vi "about status.vi"(8 "error in (no error)":errorcluster, 11 "Connection Refnum":T1) -> (0 "error out":errorcluster, 3 "Keys":T2)   [LabVIEW 2011]
uses:
  ITK EXT/utils/keyedarr.llb/Keyed Array.ctl
  Summitek EXT/ODBC/SQL Controls/Connection Refnum.ctl
  server/database/Users/User Record.ctl
  server/server lib/Spartan Version.vi
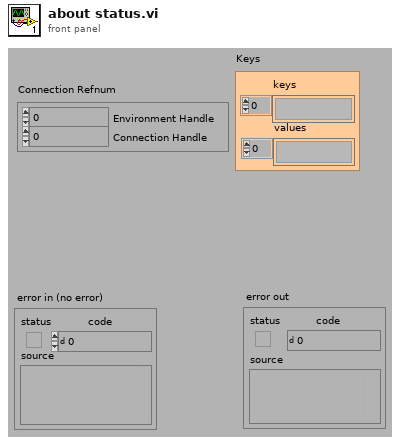
[diagram p1: front panel]
types:
  T1 = typedef "Connection Refnum.ctl" = cluster{"Environment Handle":i32, "Connection Handle":i32}
  T2 = typedef "Keyed Array.ctl" = cluster{"keys":string[], "values":string[]}
  T3 = typedef "User Record.ctl" = cluster{"ixUser":i32, "sxUsername":string, "sLastName":string, "sFirstName":string, "sEmail":string, "sPassword":string, "tLoginTime":timestamp, "sLoginComputer":string, "fAdministrator":bool, "fRunSequences":bool, "fModifySequences":bool, "fRunScenarios":bool, "fModifyScenarios":bool, "fModifyTemplates":bool, "fModifyUsers":bool, "fModifyStations":bool, "fModifyFields":bool}
  T4 = typedef "OGAB Version.ctl" = cluster{"Version":string, "Build Number":u32, "Build Date/Time":dbl}
  T5 = cluster{"Index Size, bytes":i64, "Index Date":dbl, "Test Files":i32, "Test Runs":i32}
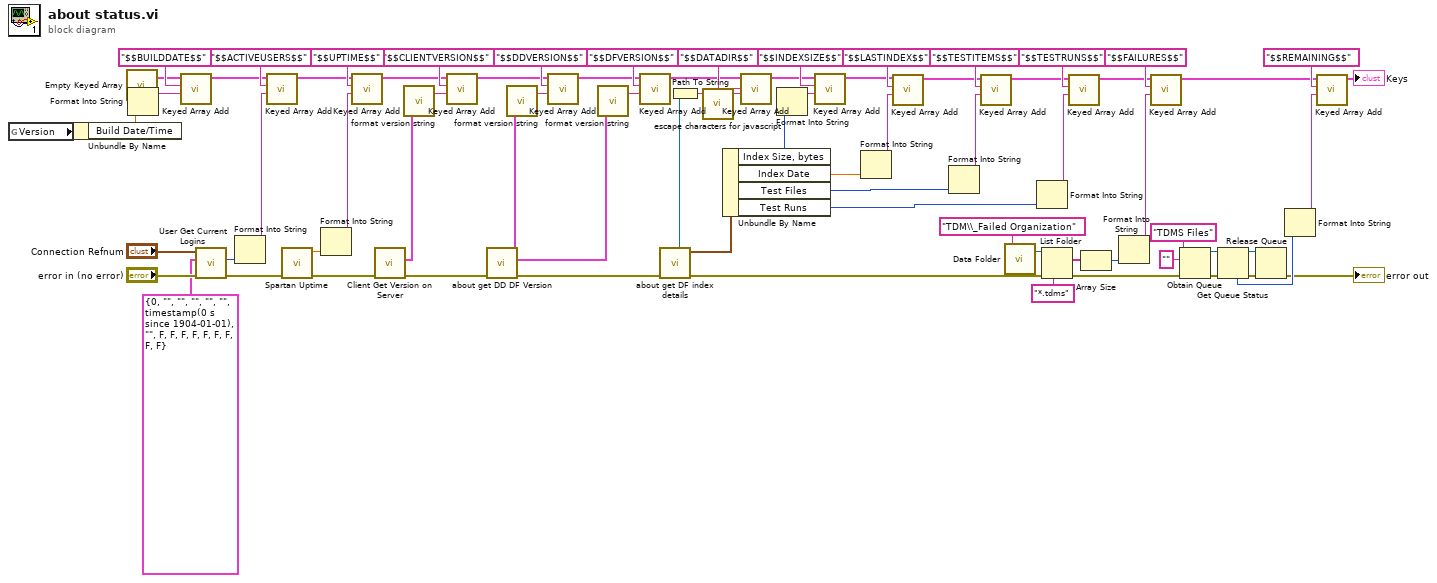
[diagram p0: block diagram]
diagram:
  n1 = global read "Spartan Version.vi" "Version"() -> (w32:T4)
  n2 = Unbundle By Name(w32) -> ("Build Date/Time"=w75:dbl)
  n3 = call "Empty Keyed Array.vi"() -> ("empty keyed array"=w25:T2)  [unwired: 3 out]
  n4 = Format Into String(w75) -> (resulting string=w74:string)  [unwired: 3 in, 1 out]
  n5 = call "Keyed Array Add.vi"("value"=w74, "key"="$$BUILDDATE$$" ("Template (\"\")"), "array in"=w25) -> ("array out"=w24:T2)  [unwired: 1 in, 3 out]
  n6 = call "User Get Current Logins.vi"("error in (no error)"="error in (no error)", "Current User (none)"=T3 {"ixUser"=0, "sxUsername"="", "sLastName"="", "sFirstName"="", "sEmail"="", "sPassword"="", "tLoginTime"=timestamp(0 s since 1904-01-01), "sLoginComputer"="", "fAdministrator"=FALSE, "fRunSequences"=FALSE, "fModifySequences"=FALSE, "fRunScenarios"=FALSE, "fModifyScenarios"=FALSE, "fModifyTemplates"=FALSE, "fModifyUsers"=FALSE, "fModifyStations"=FALSE, "fModifyFields"=FALSE}, "Connection Refnum"="Connection Refnum") -> ("error out"=w35:errorcluster, "Seats in Use"=w39:i32)  [unwired: 7 out]
  n7 = Format Into String(w39) -> (resulting string=w40:string)  [unwired: 3 in, 1 out]
  n8 = call "Keyed Array Add.vi"("value"=w40, "key"="$$ACTIVEUSERS$$" ("Template (\"\")"), "array in"=w24) -> ("array out"=w41:T2)  [unwired: 1 in, 3 out]
  n9 = call "Spartan Uptime.vi"("error in (no error)"=w35) -> ("error out"=w34:errorcluster, "Uptime"=w33:dbl)  [unwired: 9 in]
  n10 = Format Into String(w33) -> (resulting string=w43:string)  [unwired: 3 in, 1 out]
  n11 = call "Keyed Array Add.vi"("value"=w43, "key"="$$UPTIME$$" ("Template (\"\")"), "array in"=w41) -> ("array out"=w23:T2)  [unwired: 1 in, 3 out]
  n12 = call "Client Get Version on Server.vi"("error in (no error)"=w34) -> ("error out"=w57:errorcluster, "Version"=w63:T4)  [unwired: 9 out]
  n13 = call "format version string.vi"("Version"=w63) -> ("Version String"=w62:string)  [unwired: 2 out]
  n14 = call "Keyed Array Add.vi"("value"=w62, "key"="$$CLIENTVERSION$$" ("Template (\"\")"), "array in"=w23) -> ("array out"=w71:T2)  [unwired: 1 in, 3 out]
  n15 = call "about get DD DF Version.vi"("error in (no error)"=w57) -> ("error out"=w56:errorcluster, "DF Version"=w53:T4, "DD Version"=w55:T4)  [unwired: 8 out]
  n16 = call "format version string.vi"("Version"=w55) -> ("Version String"=w54:string)  [unwired: 2 out]
  n17 = call "Keyed Array Add.vi"("value"=w54, "key"="$$DDVERSION$$" ("Template (\"\")"), "array in"=w71) -> ("array out"=w69:T2)  [unwired: 1 in, 3 out]
  n18 = call "format version string.vi"("Version"=w53) -> ("Version String"=w52:string)  [unwired: 2 out]
  n19 = call "Keyed Array Add.vi"("value"=w52, "key"="$$DFVERSION$$" ("Template (\"\")"), "array in"=w69) -> ("array out"=w28:T2)  [unwired: 1 in, 3 out]
  n20 = call "about get DF index details.vi"("error in (no error)"=w56) -> ("error out"=w11:errorcluster, "Index Details"=w49:T5, "Data Repository Path"=w26:path)  [unwired: 8 out]
  n21 = Path To String(path=w26) -> (string=w30:string)
  n22 = call "escape characters for javascript.vi"("String (\"\")"=w30) -> ("escaped String"=w29:string)  [unwired: 4 in]
  n23 = Unbundle By Name(w49) -> ("Index Size, bytes"=w48:i64, "Index Date"=w47:dbl, "Test Files"=w46:i32, "Test Runs"=w45:i32)
  n24 = call "Keyed Array Add.vi"("value"=w29, "key"="$$DATADIR$$" ("Template (\"\")"), "array in"=w28) -> ("array out"=w27:T2)  [unwired: 1 in, 3 out]
  n25 = Format Into String(w48) -> (resulting string=w61:string)  [unwired: 3 in, 1 out]
  n26 = call "Keyed Array Add.vi"("value"=w61, "key"="$$INDEXSIZE$$" ("Template (\"\")"), "array in"=w27) -> ("array out"=w51:T2)  [unwired: 1 in, 3 out]
  n27 = Format Into String(w47) -> (resulting string=w58:string)  [unwired: 3 in, 1 out]
  n28 = call "Keyed Array Add.vi"("value"=w58, "key"="$$LASTINDEX$$" ("Template (\"\")"), "array in"=w51) -> ("array out"=w50:T2)  [unwired: 1 in, 3 out]
  n29 = Format Into String(w46) -> (resulting string=w60:string)  [unwired: 3 in, 1 out]
  n30 = call "Keyed Array Add.vi"("value"=w60, "key"="$$TESTITEMS$$" ("Template (\"\")"), "array in"=w50) -> ("array out"=w64:T2)  [unwired: 1 in, 3 out]
  n31 = call "Data Folder.vi"("Relative Path (\"\" - Folder)"="TDM\\_Failed Organization" ("Relative Path (\"\" - Folder)")) -> ("Data Folder"=w7:path)  [unwired: 2 in]
  n32 = Format Into String(w45) -> (resulting string=w59:string)  [unwired: 3 in, 1 out]
  n33 = List Folder(path=w7, pattern="*.tdms", error in=w11) -> (filenames=w6:string[], error out=w10:errorcluster)  [unwired: 1 in, 2 out]
  n34 = call "Keyed Array Add.vi"("value"=w59, "key"="$$TESTRUNS$$" ("Template (\"\")"), "array in"=w64) -> ("array out"=w18:T2)  [unwired: 1 in, 3 out]
  n35 = Array Size(array=w6) -> (size(s)=w5:i32)
  n36 = Format Into String(w5) -> (resulting string=w4:string)  [unwired: 3 in, 1 out]
  n37 = call "Keyed Array Add.vi"("value"=w4, "key"="$$FAILURES$$" ("Template (\"\")"), "array in"=w18) -> ("array out"=w20:T2)  [unwired: 1 in, 3 out]
  n38 = Obtain Queue(name (unnamed)="TDMS Files", element data type="", error in (no error)=w10) -> (queue out=w12:refnum<queue>, error out=w15:errorcluster)  [unwired: 2 in, 1 out]
  n39 = Get Queue Status(queue=w12, error in (no error)=w15) -> (queue out=w13:refnum<queue>, error out=w14:errorcluster, # elements in queue=w3:i32)  [unwired: 1 in, 5 out]
  n40 = Release Queue(queue=w13, error in (no error)=w14) -> (error out=→"error out":errorcluster)  [unwired: 1 in, 2 out]
  n41 = Format Into String(w3) -> (resulting string=w19:string)  [unwired: 3 in, 1 out]
  n42 = call "Keyed Array Add.vi"("value"=w19, "key"="$$REMAINING$$" ("Template (\"\")"), "array in"=w20) -> ("array out"=→"Keys":T2)  [unwired: 1 in, 3 out]
